vi "Global 1.vi"() -> ()   [LabVIEW 2014]
panel:
  out "time0":dbl
  out "DataFileWait":bool caption="Run test"
  out "DataADCNumber":u32
  in  "PixelNumber":u32[](array[numeric])=[10016] format="%0d"
  out "wait data":u16
  in  "Switch channel":bool[](array[boolean])=[TRUE, TRUE, TRUE, TRUE, TRUE, TRUE, TRUE, TRUE]
  out "SetupString":string
  out "ReadbackDone":bool caption="Run test"
  out "readbackArray":u32[](array[numeric]) format="%x"
  in  "LogFile":path=path "C:/DAMIC/DAMIC-LTC/Data/log.txt"
  in  "TSfile folder":path=path "C:/Users/lpnhe/Desktop/Labview/damic/DAMIC_TIMESLICE" caption="Path to user TS"
  in  "Output aspic file folder":path=path "C:/Users/lpnhe/Desktop/Labview/damic/DAMIC-LTC/Data"
  in  "LogDirectory":path=path "C:/DAMIC/DAMIC-LTC/Data"
  in  "TS file":string="C:\\Users\\lpnhe\\Desktop\\Labview\\damic\\DAMIC-LTC\\DamicLTC-seul-Essai.txt"
  out "dataBlockArray1":string[](array[string])
  in  "filenamesniff":string
  out "dataADCArray":i32[](array[numeric]) format="%x"
  in  "aspicdata2Default":u32[](array[numeric])=[196608, 0, 0, 0, 0, 0] format="%07x"
  in  "aspic2data":u32[](array[numeric])=[2863311530, 3149642683, 3435973836, 3722304989, 4008636142, 4294967295, 10, 10, 10, 10, 10, 10, 10, 10, 10, 10, 10, 10, 10, 10, 10, 10, 10, 10, 10, 10, 10, 10, 10, 10, 10, 10] format="%07x"
  out "UDPHaveData":bool caption="Run test"
  in  "aspicdataDefault":u32[](array[numeric])=[8388625, 8454144, 8519680] format="%07x"
  in  "aspicdata":u32[](array[numeric])=[2863311530, 3149642683, 3435973836, 3722304989, 4008636142, 4294967295, 10, 10, 10, 10, 10, 10, 10, 10, 10, 10, 10, 10, 10, 10, 10, 10, 10, 10, 10, 10, 10, 10, 10, 10, 10, 10] format="%07x"
  in  "filename":string
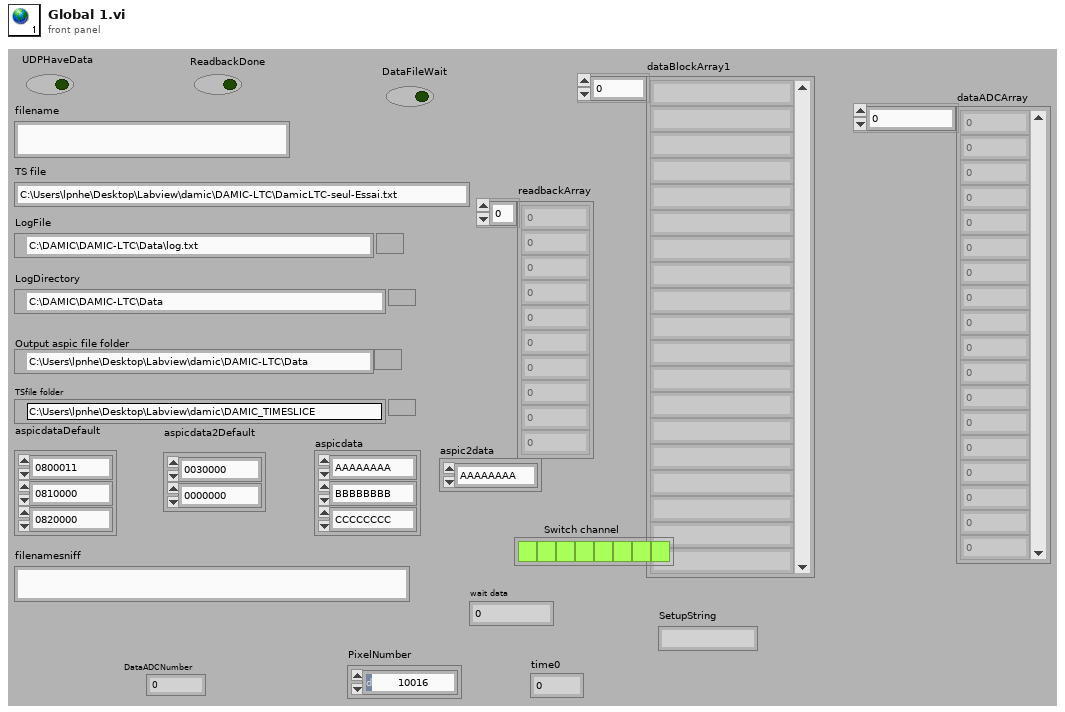
[diagram p1: front panel]
diagram:
